vi "client.vi"(8 "error in":errorcluster, 9 "subscriptions queue":refnum<queue>, 10 "nats connection":T1={"connection ID"=refnum, "server INFO"="", "timeout ms"=5000, "verbose?"=FALSE, "server headers?"=FALSE, "client headers?"=FALSE}, 11 "async stop notifier":refnum<notifier>) -> (0 "error out":errorcluster)   [LabVIEW 2024, in "NATS Client.lvlib" / "NATS Client.lvclass"]
doc: "Reads a message from the NATS server."
uses:
  NATS Client.lvclass
  NATS Client.lvclass/NATS Client.ctl
  NATS Core.lvlib
  NATS Subscription/NATS Subscription.lvclass
  Controls/nats connection.ctl
  subscription actions.ctl
  subscription queue.ctl
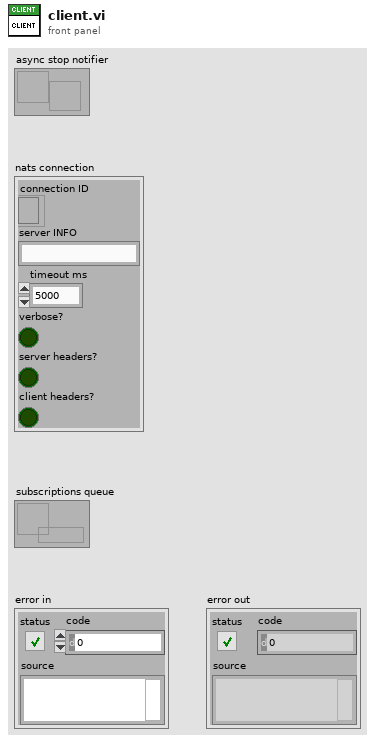
[diagram p1: front panel]
types:
  T1 = typedef "NATS Core.lvlib/nats connection.ctl" = cluster{"connection ID":refnum<k5>, "server INFO":string, "timeout ms":i32, "verbose?":bool, "server headers?":bool, "client headers?":bool}
  T2 = map{string, refnum<class "NATS Subscription.lvclass">}
  T3 = typedef "NATS Client.lvlib/NATS Client.lvclass/subscription queue.ctl" = cluster{"action":T4, "subscription":refnum<class "NATS Subscription.lvclass">}
  T4 = typedef "NATS Client.lvlib/NATS Client.lvclass/subscription actions.ctl" = enum16{"sub", "unsub"}
  T5 = typedef "NATS Core.lvlib/nats message.ctl" = cluster{"subject":string, "payload":string, "sub id":string, "reply-to":string, "headers":string, "type":T6, "received":timestamp}
  T6 = typedef "NATS Core.lvlib/msg type.ctl" = enum16{"Undefined", "MSG", "HMSG", "+OK", "PING", "PONG", "-ERR", "INFO"}
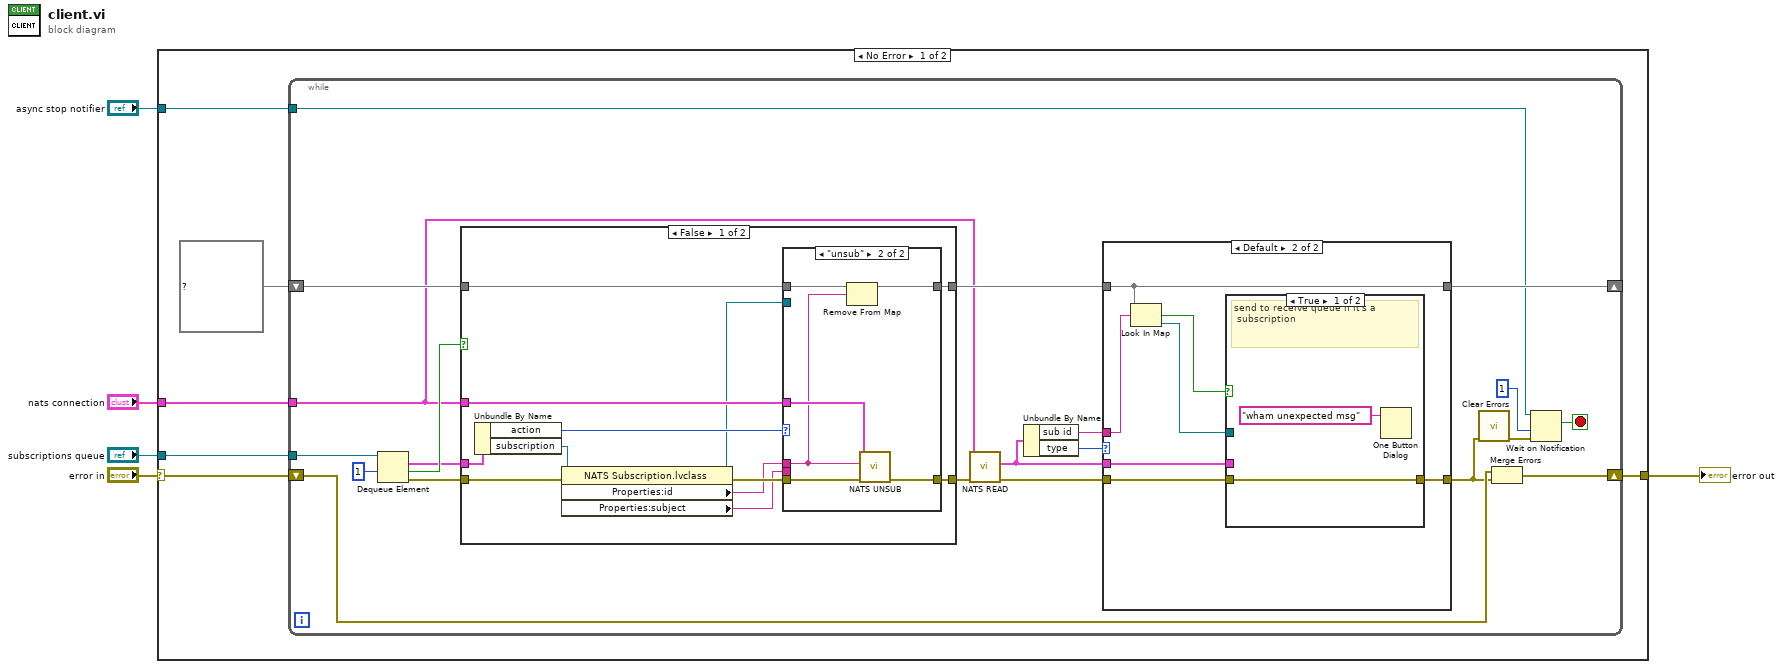
[diagram p0: block diagram]
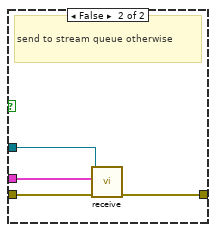
[diagram p3: hidden frame]
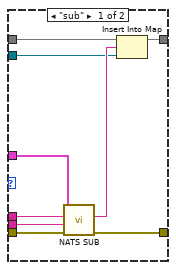
[diagram p4: hidden frame]
diagram:
  n1 = case shown="No Error" "error in" {
    selector: "error in" -> [w10 w77]
    tunnel: [w11 w77] -> w4
    tunnel: "async stop notifier" -> [w8 _]
    tunnel: "nats connection" -> [w7 _]
    tunnel: "subscriptions queue" -> [w6 _]
    frame No Error {
      n2 = while {
        tunnel: w7 -> [w14]
        tunnel: w6 -> [w25]
        shift-right: [w23] -> _
        shift-left: T2 {} ("map") -> [w16]
        tunnel: w8 -> [w20]
        shift-right: [w30] -> w11
        shift-left: w10 -> [w31]
        stop <- w19 stop-if-true
        n3 = Dequeue Element(queue=w25, timeout in ms (-1)=1) -> (element=w13:T3, timed out?=w17:bool, error out=w27:errorcluster)  [unwired: 1 in, 1 out]
        n4 = case shown="False" w17 {
          tunnel: w16 -> [w56 w75]
          tunnel: [w55 w75] -> w15
          tunnel: w27 -> [w59 w76]
          tunnel: w14 -> [w54 _]
          tunnel: [w58 w76] -> w26
          tunnel: w13 -> [w50 _]
          frame False {
            n5 = Unbundle By Name(w50) -> ("action"=w49:T4, "subscription"=w51:refnum<class "NATS Subscription.lvclass">)
            n6 = property class="NATS Subscription.lvclass"(reference=w51, error in=w59) -> (reference out=w48:refnum<class "NATS Subscription.lvclass">, error out=w57:errorcluster, "Properties:id"=w52:string, "Properties:subject"=w53:string)
            n7 = case shown="\"unsub\"" w49 {
              tunnel: w56 -> [w66 w71]
              tunnel: [w65 w72] -> w55
              tunnel: w57 -> [w68 w74]
              tunnel: w54 -> [w64 w70]
              tunnel: [w67 w73] -> w58
              tunnel: w53 -> [w62 _]
              tunnel: w52 -> [w61 w69]
              tunnel: w48 -> [w60 _]
              frame "sub" {
                n8 = call "NATS SUB.vi"("error in"=w68, "subject"=w62, "sub id"=w61, "nats connection in"=w64) -> ("error out"=w67:errorcluster, "dup sub id"=w63:string)  [unwired: 5 in, 1 out]
                n9 = Insert Into Map(map in=w66, key=w63, value=w60) -> (map out=w65:T2)  [unwired: 2 out]
              }
              frame "unsub" {
                n10 = Remove From Map(10:w69, 11:w71) -> (3:w72:T2)  [unwired: 2 out]
                n11 = call "NATS UNSUB.vi"("error in"=w74, "sub id"=w69, "nats connection in"=w70) -> ("error out"=w73:errorcluster)  [unwired: 7 in, 1 out]
              }
            }
          }
          frame True {
          }
        }
        n12 = call "NATS READ.vi"("error in"=w26, "nats connection in"=w14) -> ("error out"=w32:errorcluster, "nats message"=w12:T5)  [unwired: 6 in, 2 out]
        n13 = Unbundle By Name(w12) -> ("sub id"=w24:string, "type"=w18:T6)
        n14 = case shown="Default" w18 {
          tunnel: w32 -> [w34 w41]
          tunnel: w24 -> [_ w39]
          tunnel: w15 -> [w33 w38]
          tunnel: [w33 w38] -> w23
          tunnel: [w34 w40] -> w29
          tunnel: w12 -> [_ w36]
          frame "Undefined" {
          }
          frame Default {
            n15 = Look In Map(map=w38, key=w39) -> (key not found?=w37:bool, value=w35:refnum<class "NATS Subscription.lvclass">)  [unwired: 1 in]
            n16 = case shown="True" w37 {
              tunnel: w41 -> [w43 w47]
              tunnel: [w43 w46] -> w40
              tunnel: w36 -> [_ w44]
              tunnel: w35 -> [_ w45]
              frame True {
                # "send to receive queue if it's a\n subscription"
                n17 = One Button Dialog(message="wham unexpected msg") -> ()  [unwired: 1 in, 1 out]
              }
              frame False {
                # "send to stream queue otherwise"
                n18 = call-dynamic "receive.vi"("error in"=w47, "nats message"=w44, "NATS Subscriber in"=w45) -> ("error out"=w46:errorcluster)  [unwired: 7 in, 1 out]
              }
            }
          }
        }
        n19 = call <vilib>:"Clear Errors.vi"("error in (no error)"=w29) -> ("error out"=w28:errorcluster)  [unwired: 5 in, 1 out]
        n20 = Merge Errors(w31, w29) -> (w30:errorcluster)
        n21 = Wait on Notification(notifier=w20, timeout in ms (-1)=1, error in (no error)=w28) -> (notification=w19:bool)  [unwired: 1 in, 3 out]
      }
    }
    frame Error {
    }
  }
  "error out" <- w4
